vi "Read Reference.vi"(8 "error in (no error)":errorcluster, 11 "PmuAnalysis in":refnum<class "PmuAnalysis.lvclass">) -> (0 "error out":errorcluster, 2 "PmuReport":T1 {"Synx" format="%#_4g"; "Timestamp" format="%.6f"}, 3 "PmuAnalysis out":refnum<class "PmuAnalysis.lvclass">)   [LabVIEW 2014, in "AnalysisPlugins.lvlib" / "PmuAnalysis.lvclass"]
uses:
  PmuAnalysis.lvclass
  Typedefs/PmuData.ctl
  PmuAnalysis.lvclass/PmuAnalysis.ctl
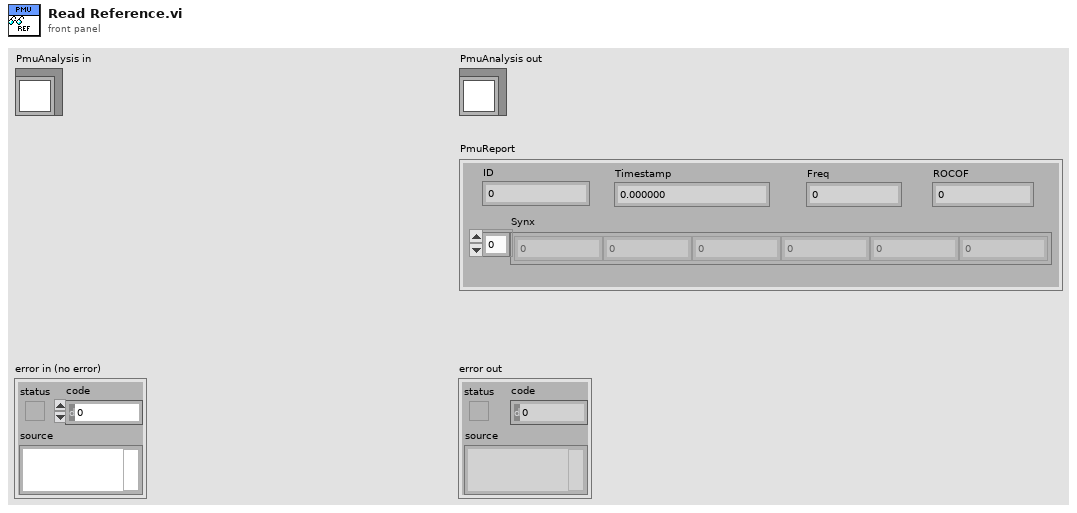
[diagram p1: front panel]
types:
  T1 = typedef "AnalysisPlugins.lvlib/PmuAnalysis.lvclass/PmuData.ctl" = cluster{"Timestamp":dbl, "Synx":cdb[], "Freq":dbl, "ROCOF":dbl, "ID":i16}
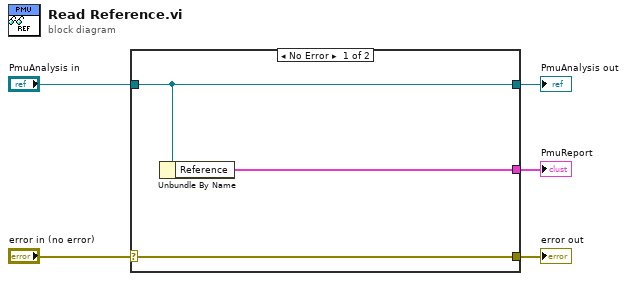
[diagram p0: block diagram]
diagram:
  n1 = case shown="No Error" "error in (no error)" {
    selector: "error in (no error)" -> [w8 w9]
    tunnel: [w8 w9] -> w4
    tunnel: [w7 w10] -> w2
    tunnel: "PmuAnalysis in" -> [w7 w10]
    tunnel: [w6 _] -> w1
    frame No Error {
      n2 = Unbundle By Name(w7) -> ("Reference"=w6:T1)
    }
    frame Error {
    }
  }
  "error out" <- w4
  "PmuAnalysis out" <- w2
  "PmuReport" <- w1
